vi "Sub02_PixmapBin.vi"(8 "error in (no error)":errorcluster, 9 "String":string, 10 "path in":path) -> (0 "error out":errorcluster, 5 "new picture":picture)   [LabVIEW 2019]
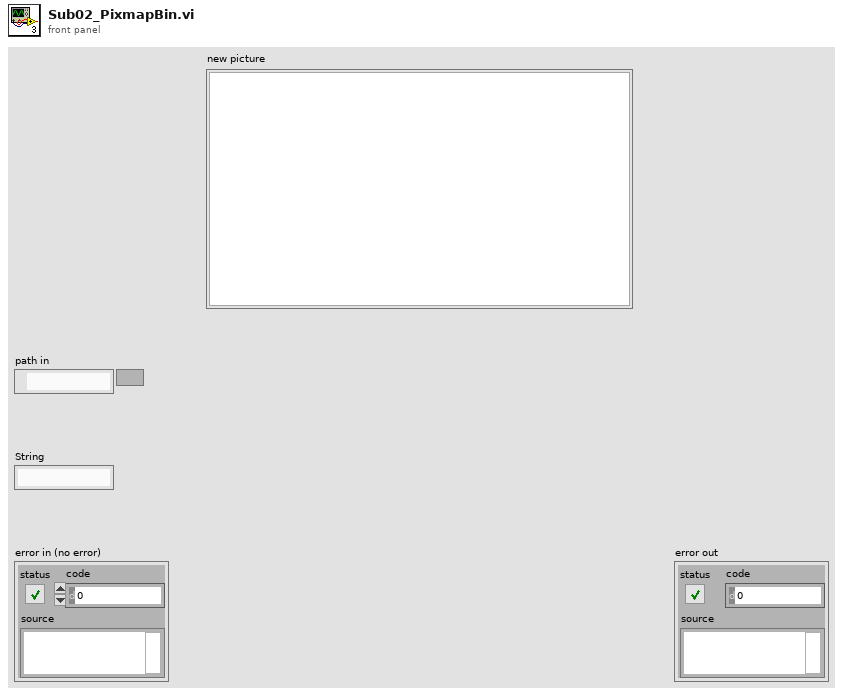
[diagram p1: front panel]
types:
  T1 = enum16{"big-endian, network order", "native, host order", "little-endian"}
  T2 = typedef "imagedata.ctl" = cluster{"image type":i32, "image depth":i32, "image":u8[], "mask":u8[], "colors":u32[], "Rectangle":cluster{"left":i16, "top":i16, "right":i16, "bottom":i16}}
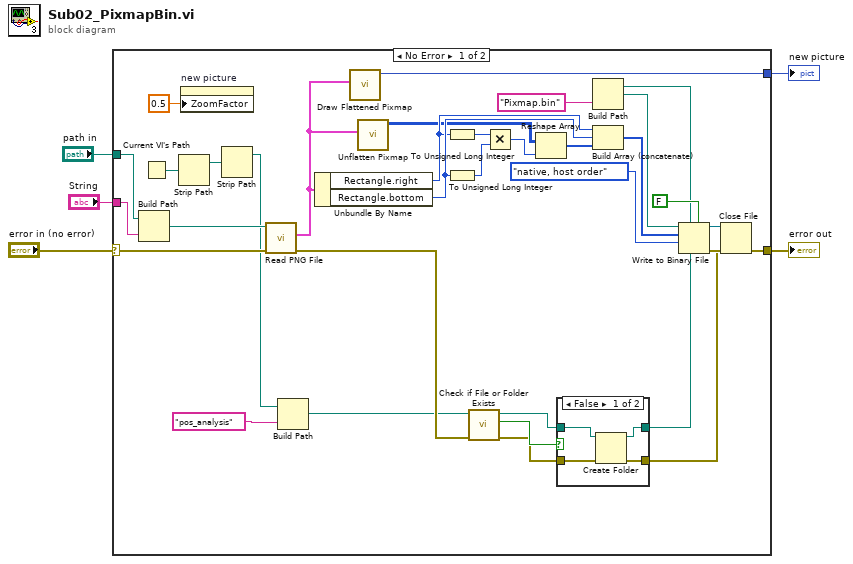
[diagram p0: block diagram]
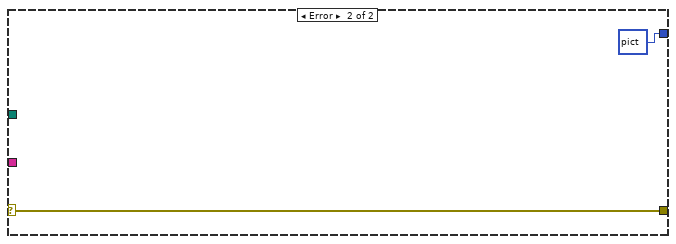
[diagram p3: hidden frame]
diagram:
  n1 = case shown="No Error" "error in (no error)" {
    selector: "error in (no error)" -> [w18 w45]
    tunnel: [w27 w45] -> w5
    tunnel: "String" -> [w24 _]
    tunnel: "path in" -> [w23 _]
    tunnel: [w21 picture data[5B] ("new picture")] -> w2
    frame No Error {
      n2 = Build Path(base path=w23, name or relative path=w24) -> (appended path=w25:path)
      n3 = Current VI's Path() -> (path=w20:path)
      n4 = Strip Path(path=w20) -> (stripped path=w17:path)  [unwired: 1 out]
      n5 = property on="new picture" class="Pict"("ZoomFactor"=sgl 0.5 ("Zoom Factor")) -> ()  [unwired: 2 in, 2 out]
      n6 = Strip Path(path=w17) -> (stripped path=w16:path)  [unwired: 1 out]
      n7 = call <vilib>:"Read PNG File.vi"("error in (no error)"=w18, "path to PNG file"=w25) -> ("error out"=w12:errorcluster, "image data"=w22:T2)  [unwired: 7 in, 1 out]
      n8 = Build Path(base path=w16, name or relative path="pos_analysis") -> (appended path=w9:path)
      n9 = Unbundle By Name(w22) -> ("Rectangle.right"=w32:i16, "Rectangle.bottom"=w33:i16)
      n10 = call <vilib>:"Draw Flattened Pixmap.vi"("image data"=w22) -> ("new picture"=w21:picture)  [unwired: 8 in]
      n11 = call <vilib>:"Unflatten Pixmap.vi"("image data"=w22) -> ("24-bit pixmap"=w26:u32[][])  [unwired: 4 in, 6 out]
      n12 = To Unsigned Long Integer(number=w32) -> (unsigned 32bit integer=w28:u32)
      n13 = To Unsigned Long Integer(number=w33) -> (unsigned 32bit integer=w29:u32)
      n14 = call <vilib>:"Check if File or Folder Exists.vi"("error in (no error)"=w12, "path"=w9) -> ("error out"=w11:errorcluster, "file or folder exists?"=w13:bool, "dup path"=w8:path)  [unwired: 7 in]
      n15 = Multiply(x=w28, y=w29) -> (x*y=w30:u32)
      n16 = Reshape Array(w26, w30) -> (w31:u32[])
      n17 = case shown="False" w13 {
        tunnel: w11 -> [w42 w44]
        tunnel: w8 -> [w41 w43]
        tunnel: [w40 w44] -> w10
        tunnel: [w39 w43] -> w6
        frame False {
          n18 = Create Folder(path (use dialog)=w41, error in=w42) -> (created path=w39:path, error out=w40:errorcluster)  [unwired: 1 in, 1 out]
        }
        frame True {
        }
      }
      n19 = Build Path(base path=w6, name or relative path="Pixmap.bin") -> (appended path=w7:path)
      n20 = Build Array (concatenate)(w32, w33, w31) -> (w34:u32[])
      n21 = Write to Binary File(file (use dialog)=w7, data=w34, error in=w10, 5:FALSE ("prepend array or string size? (T)"), 9:T1."native, host order" ("byte order (0:big-endian, network order)")) -> (refnum out=w38:refnum<file>, error out=w37:errorcluster)  [unwired: 1 in, 1 out]
      n22 = Close File(refnum=w38, error in=w37) -> (error out=w27:errorcluster)  [unwired: 1 out]
    }
    frame Error {
    }
  }
  "error out" <- w5
  "new picture" <- w2
